vi "4024_output.vi"(0 "Address":T1, 3 "Set to:":dbl min=-10.0 max=20.0 format="%.3f", 4 "Channel Name":string) -> (5 "Comment":string, 7 "Reading":dbl format="%.3f")   [LabVIEW 2020]
uses:
  ADAM Client/Sub VIs/ADAM Controls/Address.ctl
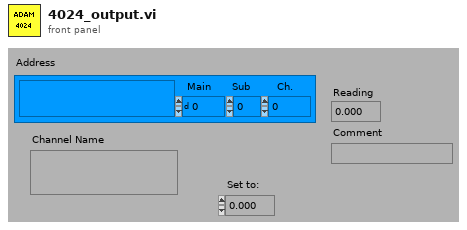
[diagram p1: front panel]
types:
  T1 = typedef "Address.ctl" = cluster{"Main":i32, "Ch.":i32, "Sub":i32, "Port Name":string}
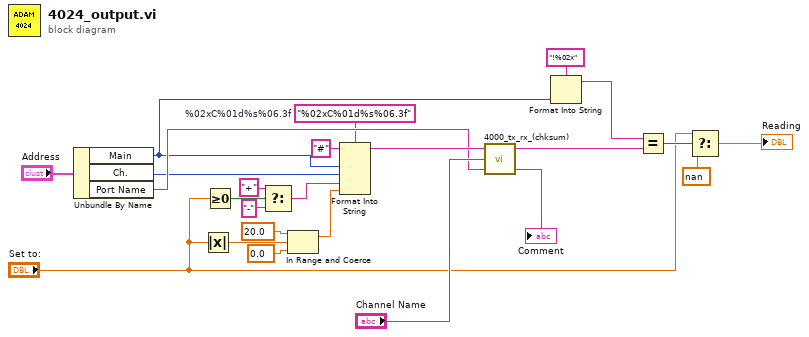
[diagram p0: block diagram]
diagram:
  w17 = "%02xC%01d%s%06.3f"  # %02xC%01d%s%06.3f
  n1 = Unbundle By Name("Address") -> ("Main"=w9:i32, "Ch."=w11:i32, "Port Name"=w18:string)
  n2 = Absolute Value(x="Set to:") -> (abs(x)=w2:dbl)
  n3 = Greater Or Equal To 0?(x="Set to:") -> (x >= 0?=w7:bool)
  n4 = Select(t="+", s=w7, f="-") -> (s? t:f=w4:string)
  n5 = In Range and Coerce(upper limit=20.0 ("Max"), x=w2, lower limit=0.0 ("Min")) -> (coerced(x)=w3:dbl)  [unwired: 1 out]
  n6 = Format Into String(format string=w17, initial string="#", w9, w11, w4, w3) -> (resulting string=w22:string)  [unwired: 1 in, 1 out]
  n7 = call "4000_tx_rx_(chksum).vi"("Write String"=w22, "Channel Name"="Channel Name", "Port Name"=w18) -> ("Read"=w21:string, "Comment out"=→"Comment":string)  [unwired: 2 in, 1 out]
  n8 = Format Into String(format string="!%02x", w9) -> (resulting string=w8:string)  [unwired: 2 in, 1 out]
  n9 = Equal?(x=w8, y=w21) -> (x = y?=w13:bool)
  n10 = Select(t="Set to:", s=w13, f=nan) -> (s? t:f=→"Reading":dbl)
